vi "Init Resources.vi"(8 "error in (no error)":errorcluster, 11 "Session in":refnum<class "Session.lvclass">) -> (0 "error out":errorcluster, 3 "Session out":refnum<class "Session.lvclass">)   [LabVIEW 2024, in "CTI.lvlib" / "Session.lvclass"]
uses:
  Session.lvclass
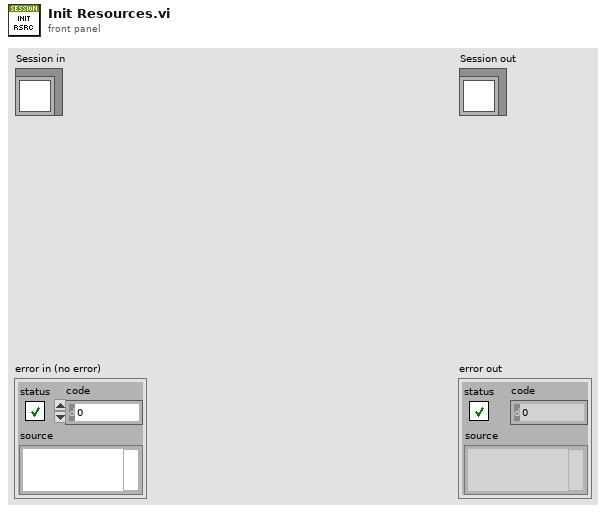
[diagram p1: front panel]
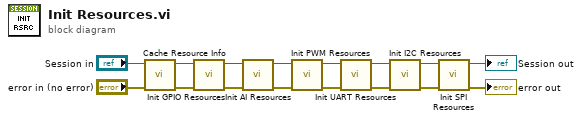
[diagram p0: block diagram]
diagram:
  n1 = call "Cache Resource Info.vi"("error in (no error)"="error in (no error)", "Session in"="Session in") -> ("error out"=w12:errorcluster, "Session out"=w10:refnum<class "Session.lvclass">)  [unwired: 8 in]
  n2 = call "Init GPIO Resources.vi"("error in (no error)"=w12, "Session in"=w10) -> ("error out"=w15:errorcluster, "Session out"=w13:refnum<class "Session.lvclass">)  [unwired: 8 in]
  n3 = call "Init AI Resources.vi"("error in (no error)"=w15, "Session in"=w13) -> ("error out"=w14:errorcluster, "Session out"=w8:refnum<class "Session.lvclass">)  [unwired: 8 in]
  n4 = call "Init PWM Resources.vi"("error in (no error)"=w14, "Session in"=w8) -> ("error out"=w9:errorcluster, "Session out"=w6:refnum<class "Session.lvclass">)  [unwired: 8 in]
  n5 = call "Init UART Resources.vi"("error in (no error)"=w9, "Session in"=w6) -> ("error out"=w7:errorcluster, "Session out"=w4:refnum<class "Session.lvclass">)  [unwired: 8 in]
  n6 = call "Init I2C Resources.vi"("error in (no error)"=w7, "Session in"=w4) -> ("error out"=w5:errorcluster, "Session out"=w2:refnum<class "Session.lvclass">)  [unwired: 8 in]
  n7 = call "Init SPI Resources.vi"("error in (no error)"=w5, "Session in"=w2) -> ("error out"=→"error out":errorcluster, "Session out"=→"Session out":refnum<class "Session.lvclass">)  [unwired: 8 in]
